vi "cleanArray.vi"(1 "Array in":string[](array[string])) -> (0 "Array out":string[](array[string]))   [LabVIEW 2013]
doc: "Removes empty array elements"
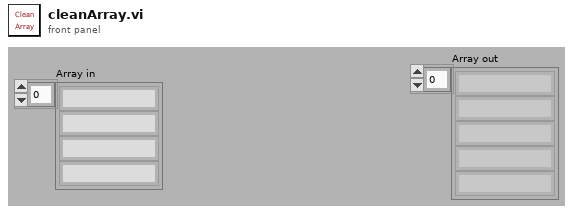
[diagram p1: front panel]
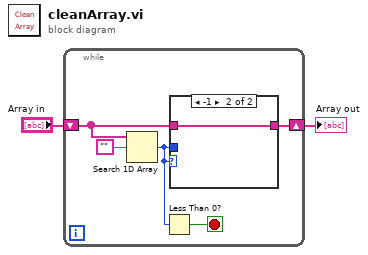
[diagram p0: block diagram]
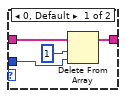
[diagram p2: hidden frame]
diagram:
  n1 = while {
    shift-right: [w3] -> w1
    shift-left: "Array in" -> [w6]
    stop <- w5 stop-if-true
    n2 = Search 1D Array(1D array=w6, element="") -> (index of element=w4:i32)  [unwired: 1 in]
    n3 = Less Than 0?(x=w4) -> (x < 0?=w5:bool)
    n4 = case shown="-1" w4 {
      tunnel: w6 -> [w11 w12]
      tunnel: w4 -> [w10 _]
      tunnel: [w8 w12] -> w3
      frame 0, Default {
        n5 = Delete From Array(array=w11, length=1, index=w10) -> (array with subset deleted=w8:string[])  [unwired: 1 out]
      }
      frame -1 {
      }
    }
  }
  "Array out" <- w1
